vi "mainClase.vi"() -> ()   [LabVIEW 2014]
uses:
  claseDB/claseDB.lvclass
panel:
  out "datosClaseDB":T1
  out "Array 2":refnum<class "claseDB.lvclass">[](array[class])
  out "Array":T2(array[cluster])
  out "datosClaseDB Objeto1":T1
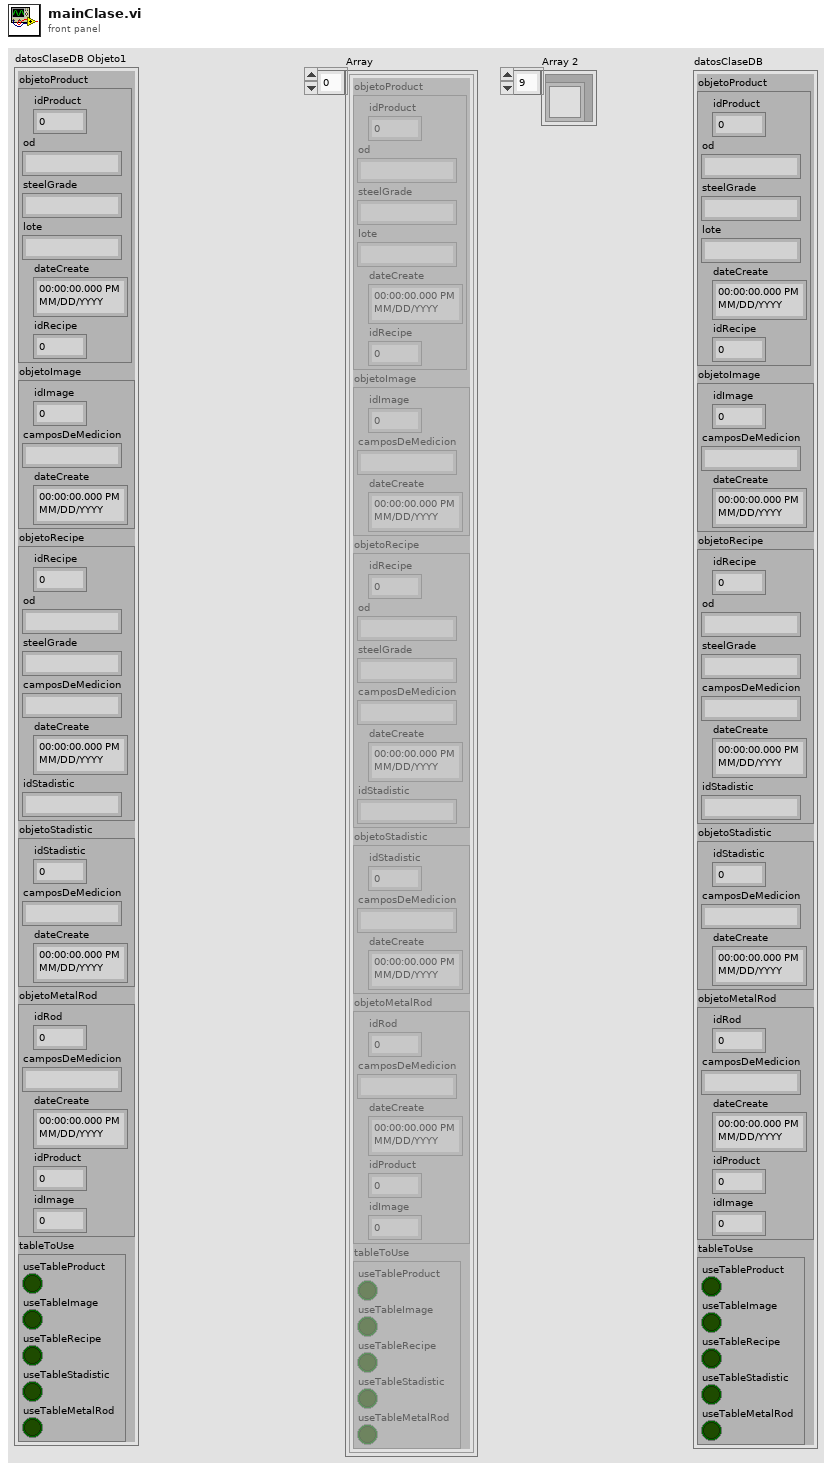
[diagram p1: front panel]
types:
  T1 = cluster{"objetoProduct":cluster{"idProduct":dbl, "od":string, "steelGrade":string, "lote":string, "dateCreate":timestamp, "idRecipe":dbl}, "objetoImage":cluster{"idImage":dbl, "camposDeMedicion":string, "dateCreate":timestamp}, "objetoRecipe":cluster{"idRecipe":dbl, "od":string, "steelGrade":string, "camposDeMedicion":string, "dateCreate":timestamp, "idStadistic":string}, "objetoStadistic":cluster{"idStadistic":dbl, "camposDeMedicion":string, "dateCreate":timestamp}, "objetoMetalRod":cluster{"idRod":dbl, "camposDeMedicion":string, "dateCreate":timestamp, "idProduct":dbl, "idImage":dbl}, "tableToUse":cluster{"useTableProduct":bool, "useTableImage":bool, "useTableRecipe":bool, "useTableStadistic":bool, "useTableMetalRod":bool}}
  T2 = cluster{"objetoProduct":cluster{"idProduct":dbl, "od":string, "steelGrade":string, "lote":string, "dateCreate":timestamp, "idRecipe":dbl}, "objetoImage":cluster{"idImage":dbl, "camposDeMedicion":string, "dateCreate":timestamp}, "objetoRecipe":cluster{"idRecipe":dbl, "od":string, "steelGrade":string, "camposDeMedicion":string, "dateCreate":timestamp, "idStadistic":string}, "objetoStadistic":cluster{"idStadistic":dbl, "camposDeMedicion":string, "dateCreate":timestamp}, "objetoMetalRod":cluster{"idRod":dbl, "camposDeMedicion":string, "dateCreate":timestamp, "idProduct":dbl, "idImage":dbl}, "tableToUse":cluster{"useTableProduct":bool, "useTableImage":bool, "useTableRecipe":bool, "useTableStadistic":bool, "useTableMetalRod":bool}}[]
  T3 = cluster{"idImage":dbl, "camposDeMedicion":string, "dateCreate":timestamp}
  T4 = cluster{"idRecipe":dbl, "od":string, "steelGrade":string, "camposDeMedicion":string, "dateCreate":timestamp, "idStadistic":string}
  T5 = cluster{"idStadistic":dbl, "camposDeMedicion":string, "dateCreate":timestamp}
  T6 = cluster{"idRod":dbl, "camposDeMedicion":string, "dateCreate":timestamp, "idProduct":dbl, "idImage":dbl}
  T7 = cluster{bool, "useTableImage":bool, "useTableRecipe":bool, "useTableStadistic":bool, "useTableMetalRod":bool}
  T8 = cluster{i32, "od":string, "steelGrade":string, "lote":string, "dateCreate":timestamp, "idRecipe":dbl}
  T9 = cluster{cluster{i32, "od":string, "steelGrade":string, "lote":string, "dateCreate":timestamp, "idRecipe":dbl}, "objetoImage":cluster{"idImage":dbl, "camposDeMedicion":string, "dateCreate":timestamp}, "objetoRecipe":cluster{"idRecipe":dbl, "od":string, "steelGrade":string, "camposDeMedicion":string, "dateCreate":timestamp, "idStadistic":string}, "objetoStadistic":cluster{"idStadistic":dbl, "camposDeMedicion":string, "dateCreate":timestamp}, "objetoMetalRod":cluster{"idRod":dbl, "camposDeMedicion":string, "dateCreate":timestamp, "idProduct":dbl, "idImage":dbl}, cluster{bool, "useTableImage":bool, "useTableRecipe":bool, "useTableStadistic":bool, "useTableMetalRod":bool}}
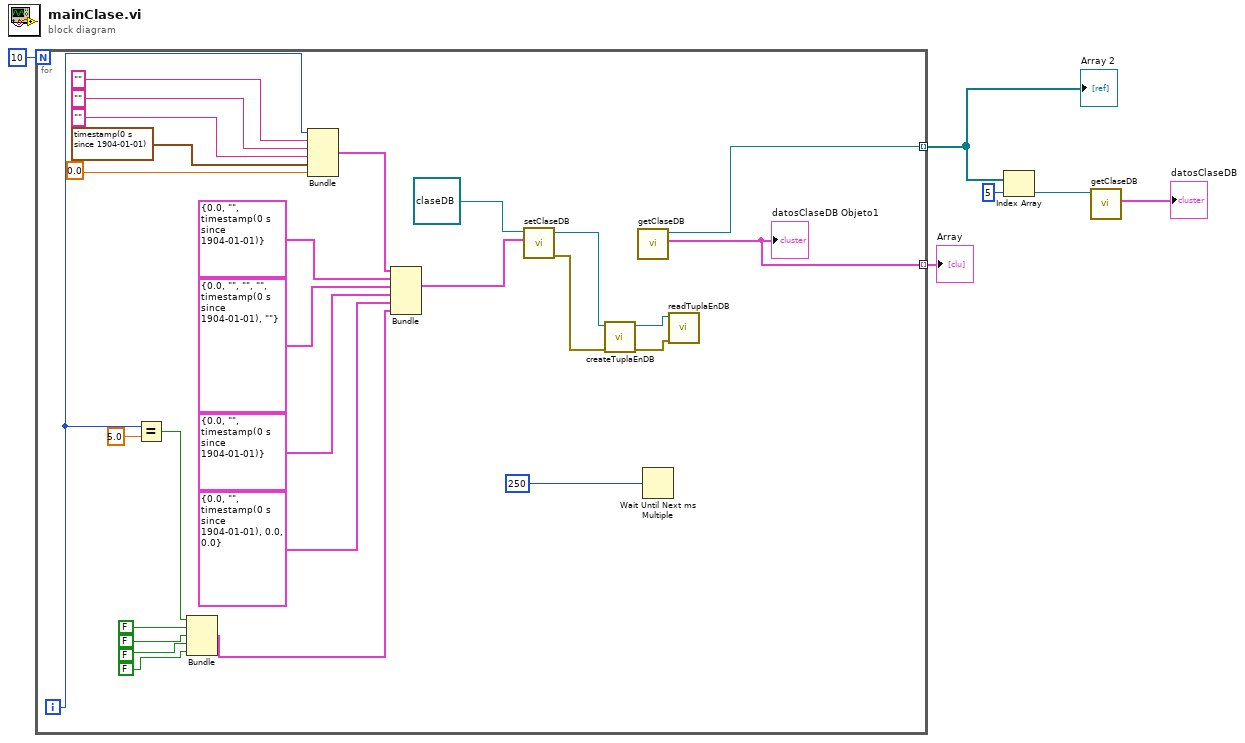
[diagram p0: block diagram]
diagram:
  n1 = for {
    N: 10 -> [_]
    tunnel: [w21] -> w6 mode=indexing
    tunnel: [w19] -> w4 mode=indexing
    i -> [w17]
    n2 = Equal?(x=w17, y=5.0) -> (x = y?=w15:bool)
    n3 = Bundle(w15, "useTableImage"=FALSE, "useTableRecipe"=FALSE, "useTableStadistic"=FALSE, "useTableMetalRod"=FALSE) -> (w16:T7)  [unwired: 1 in]
    n4 = Bundle(w17, "od"="", "steelGrade"="", "lote"="", "dateCreate"=timestamp(0 s since 1904-01-01), "idRecipe"=0.0) -> (w22:T8)  [unwired: 1 in]
    n5 = Bundle(w22, "objetoImage"=T3 {"idImage"=0.0, "camposDeMedicion"="", "dateCreate"=timestamp(0 s since 1904-01-01)}, "objetoRecipe"=T4 {"idRecipe"=0.0, "od"="", "steelGrade"="", "camposDeMedicion"="", "dateCreate"=timestamp(0 s since 1904-01-01), "idStadistic"=""}, "objetoStadistic"=T5 {"idStadistic"=0.0, "camposDeMedicion"="", "dateCreate"=timestamp(0 s since 1904-01-01)}, "objetoMetalRod"=T6 {"idRod"=0.0, "camposDeMedicion"="", "dateCreate"=timestamp(0 s since 1904-01-01), "idProduct"=0.0, "idImage"=0.0}, w16) -> (w23:T9)  [unwired: 1 in]
    n6 = call "setClaseDB.vi"("claseDBValues"=w23, "claseDB in"=refnum<class "claseDB.lvclass"> refnum ("claseDB.lvclass")) -> ("error out"=w9:errorcluster, "claseDB out"=w10:refnum<class "claseDB.lvclass">)  [unwired: 8 in]
    n7 = call "createTuplaEnDB.vi"("error in"=w9, "claseDB in"=w10) -> ("error out"=w8:errorcluster, "claseDB.lvclass"=w7:refnum<class "claseDB.lvclass">)  [unwired: 8 in]
    n8 = call "getClaseDB.vi"() -> ("datosClaseDB"=w21:T1, "claseDB.lvclass 2"=w19:refnum<class "claseDB.lvclass">)  [unwired: 9 in, 1 out]
    "datosClaseDB Objeto1" <- w21
    n9 = Wait Until Next ms Multiple(millisecond multiple=u32 250) -> ()  [unwired: 1 out]
    n10 = call "readTuplaEnDB.vi"("error in"=w8, "claseDB in"=w7) -> ()  [unwired: 8 in, 2 out]
  }
  "Array" <- w6
  "Array 2" <- w4
  n11 = Index Array(array=w4, index=5) -> (element=w2:refnum<class "claseDB.lvclass">)
  n12 = call "getClaseDB.vi"("claseDB.lvclass"=w2) -> ("datosClaseDB"=→"datosClaseDB":T1)  [unwired: 8 in, 2 out]
